vi "Read VEnum.vi"(8 "error in (no error)":errorcluster, 11 "EnumeratedVariant in":refnum<class "EnumeratedVariant.lvclass">) -> (0 "error out":errorcluster, 2 "VEnum":variant, 3 "EnumeratedVariant out":refnum<class "EnumeratedVariant.lvclass">)   [LabVIEW 2020, in "EnumeratedVariant.lvclass"]
uses:
  EnumeratedVariant.lvclass
  EnumeratedVariant.lvclass/EnumeratedVariant.ctl
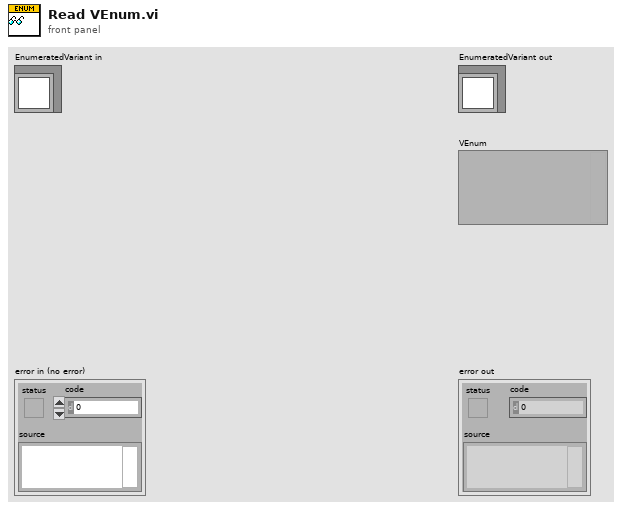
[diagram p1: front panel]
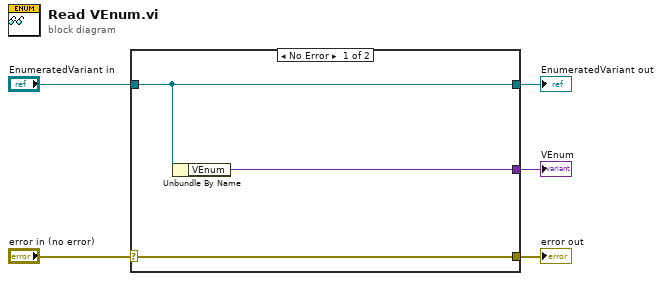
[diagram p0: block diagram]
diagram:
  n1 = case shown="No Error" "error in (no error)" {
    selector: "error in (no error)" -> [w8 w9]
    tunnel: [w8 w9] -> w4
    tunnel: [w7 w10] -> w2
    tunnel: "EnumeratedVariant in" -> [w7 w10]
    tunnel: [w6 _] -> w1
    frame No Error {
      n2 = Unbundle By Name(w7) -> ("VEnum"=w6:variant)
    }
    frame Error {
    }
  }
  "error out" <- w4
  "EnumeratedVariant out" <- w2
  "VEnum" <- w1
